vi "TimeInit.vi"(2 "error in (no error)":errorcluster, 3 "Time Card/Channels":i32[](array[numeric])=[2, 8], 4 "Data Value Reference in":refnum<data-value>) -> (0 "error out":errorcluster)   [LabVIEW 2014]
uses:
  <vilib>/MDSplus/Classes/Tree_Class/Tree.lvclass
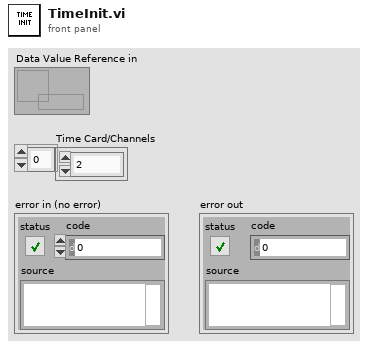
[diagram p1: front panel]
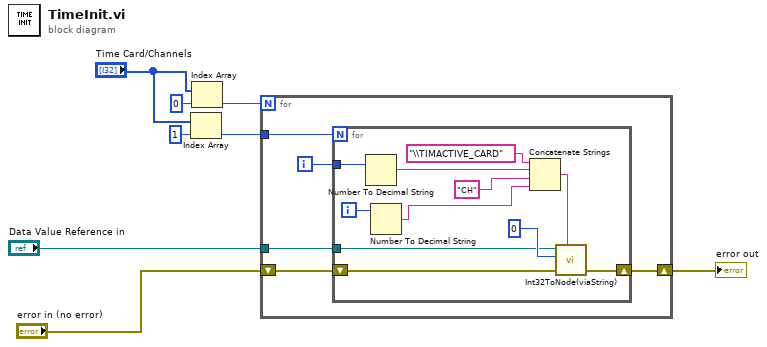
[diagram p0: block diagram]
diagram:
  n1 = Index Array(array="Time Card/Channels", index=1) -> (element=w4:i32)
  n2 = Index Array(array="Time Card/Channels", index=0) -> (element=w3:i32)
  n3 = for {
    N: w3 -> [_]
    shift-right: [w11] -> w6
    shift-left: "error in (no error)" -> [w12]
    tunnel: "Data Value Reference in" -> [w10]
    tunnel: w4 -> [w9]
    i -> [w13]
    n4 = for {
      N: w9 -> [_]
      tunnel: w13 -> [w22]
      shift-right: [w16] -> w11
      shift-left: w12 -> [w17]
      tunnel: w10 -> [w18]
      i -> [w21]
      n5 = Number To Decimal String(number=w22) -> (decimal integer string=w23:string)  [unwired: 1 in]
      n6 = Number To Decimal String(number=w21) -> (decimal integer string=w20:string)  [unwired: 1 in]
      n7 = Concatenate Strings("\\TIMACTIVE_CARD" ("string"), w23, "CH" ("string"), w20) -> (w14:string)
      n8 = call "Int32ToNode(viaString).vi"("Tree DVR in"=w18, "I32 in"=0, "error in (no error)"=w17, "NodePath"=w14) -> ("error out"=w16:errorcluster)  [unwired: 2 in, 1 out]
    }
  }
  "error out" <- w6
